vi "Queues - Init.vi"(8 "error in (no error)":errorcluster) -> (0 "error out":errorcluster, 3 "Queues":T1)   [LabVIEW 2017]
doc: "Initialize all queues in application"
uses:
  Controls/Queues.ctl
  Controller/Controls/UI CMD.ctl
  Controller/Controls/Controller CMD.ctl
  Configuration/Controls/Config CMD.ctl
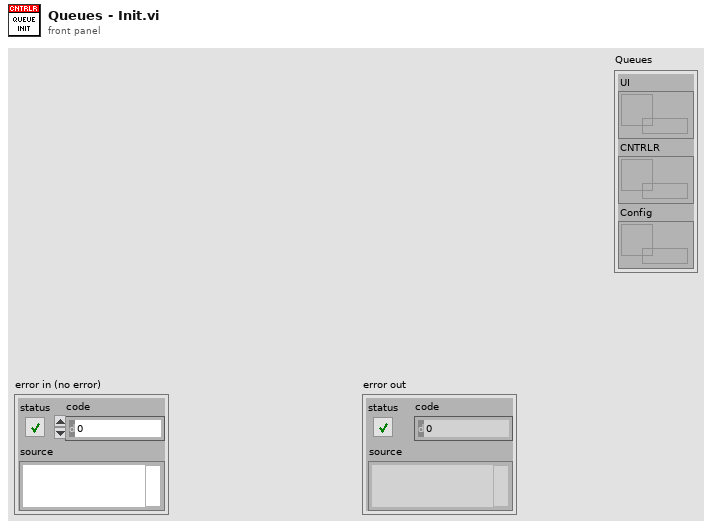
[diagram p1: front panel]
types:
  T1 = typedef "Queues.ctl" = cluster{"UI":refnum<queue>, "CNTRLR":refnum<queue>, "Config":refnum<queue>}
  T2 = typedef "Config CMD.ctl" = cluster{"CMD":enum16{"Idle", "Read", "Search", "Update", "Stop"}, "Data":variant}
  T3 = typedef "Controller CMD.ctl" = cluster{"Command":enum16{"Init"}, "Data":variant}
  T4 = typedef "UI CMD.ctl" = cluster{"Command":enum16{"Idle"}, "Data":variant}
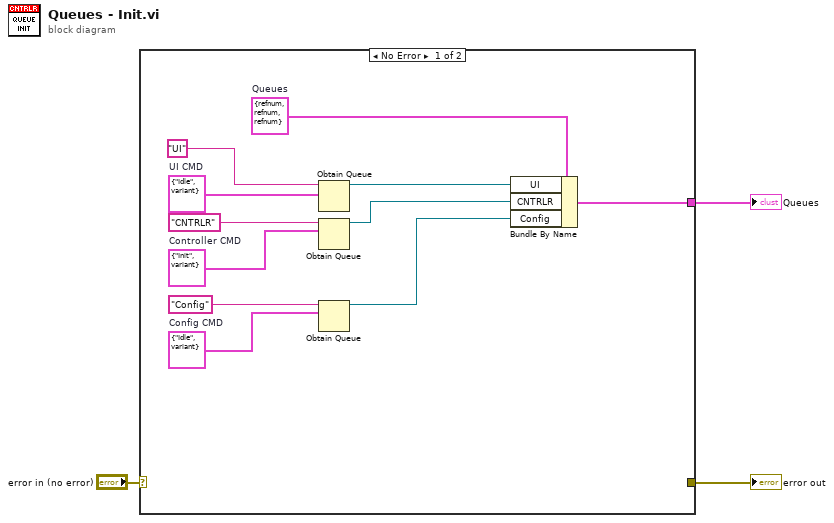
[diagram p0: block diagram]
diagram:
  n1 = case shown="No Error" "error in (no error)" {
    selector: "error in (no error)" -> [_ w15]
    tunnel: [w4 _] -> w2
    tunnel: [_ w15] -> w1
    frame No Error {
      w7 = T2 {"CMD"=enum."Idle", "Data"=variant}  # Config CMD
      w9 = T3 {"Command"=enum."Init", "Data"=variant}  # Controller CMD
      w12 = T4 {"Command"=enum."Idle", "Data"=variant}  # UI CMD
      w13 = T1 {"UI"=refnum, "CNTRLR"=refnum, "Config"=refnum}  # Queues
      n2 = Obtain Queue(name (unnamed)="UI", element data type=w12) -> (queue out=w11:refnum<queue>)  [unwired: 3 in, 2 out]
      n3 = Obtain Queue(name (unnamed)="CNTRLR", element data type=w9) -> (queue out=w6:refnum<queue>)  [unwired: 3 in, 2 out]
      n4 = Obtain Queue(name (unnamed)="Config", element data type=w7) -> (queue out=w5:refnum<queue>)  [unwired: 3 in, 2 out]
      n5 = Bundle By Name(cluster=w13, "UI"=w11, "CNTRLR"=w6, "Config"=w5) -> (w4:T1)
    }
    frame Error {
    }
  }
  "Queues" <- w2
  "error out" <- w1
